vi "WriteControl2MCU.vi"(6 "error in (no error)":errorcluster, 8 "Config":T1, 9 "Control Code":u8 format="%.0x") -> (0 "error out":errorcluster)   [LabVIEW 2016]
uses:
  Settings/Settings.ctl
  Logging/Logging Configuration.ctl
  Hardware Configuration.ctl
  <vilib>/NI Modbus.llb/MB Serial Master Query Write Multiple Coils (poly).vi
  Acquisition.lvlib
  Logging/Logging.lvlib
  Settings/Settings.lvlib
panel:
  out "Exception Code":u8 format="%.0x"
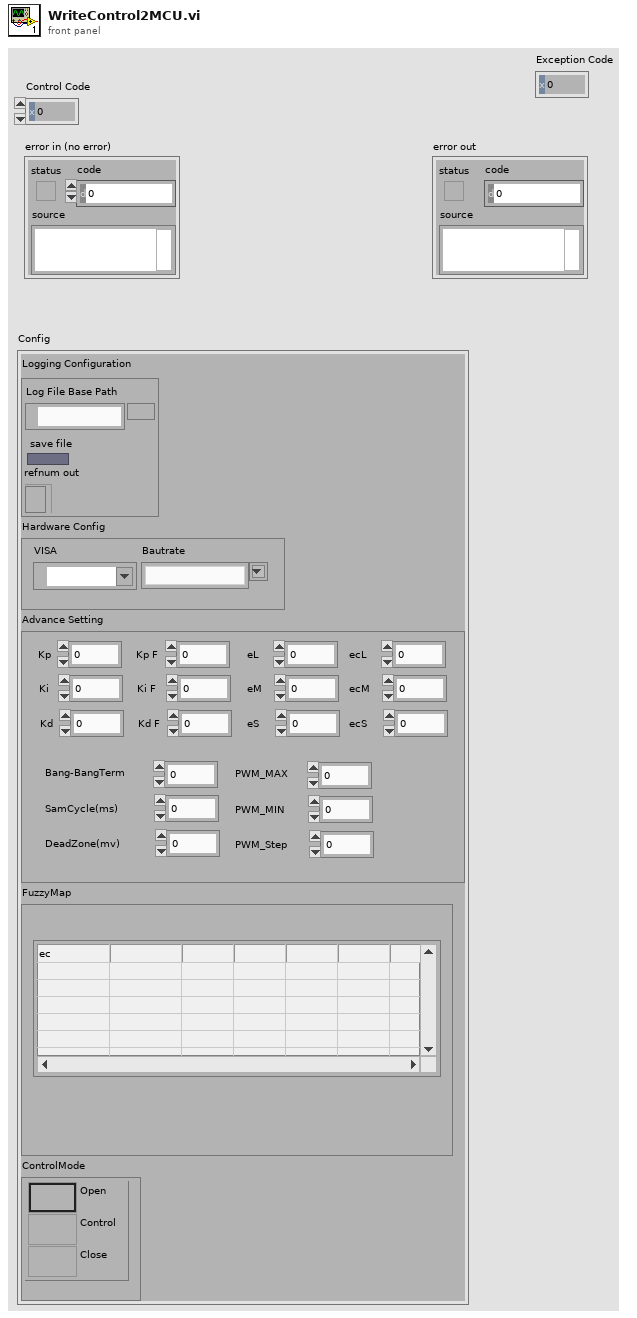
[diagram p1: front panel]
types:
  T1 = typedef "Settings.lvlib/Settings.ctl" = cluster{"Logging Configuration":T2, "Hardware Config":cluster{"Bautrate":string, "VISA":T3}, "Advance Setting":cluster{"PWM_Step":dbl, "PWM_MIN":dbl, "PWM_MAX":dbl, "DeadZone(mv)":dbl, "SamCycle(ms)":dbl, "Bang-BangTerm":dbl, "ecS":dbl, "ecM":dbl, "ecL":dbl, "eS":dbl, "eM":dbl, "eL":dbl, "Kd F":dbl, "Ki F":dbl, "Kp F":dbl, "Kd":dbl, "Ki":dbl, "Kp":dbl}, "FuzzyMap":cluster{"Table":string[][]}, "ControlMode":cluster{"Control":enum32{"1", "2", "4"}}}
  T2 = typedef "Logging.lvlib/Logging Configuration.ctl" = cluster{"Log File Base Path":path, "save file":bool, "refnum out":refnum<file>}
  T3 = typedef "Acquisition.lvlib/Hardware Configuration.ctl" = refnum<visa-resource-name>
  T4 = cluster{"Mode":enum16{"RTU", "ASCII"}, "Slave Address":u8}
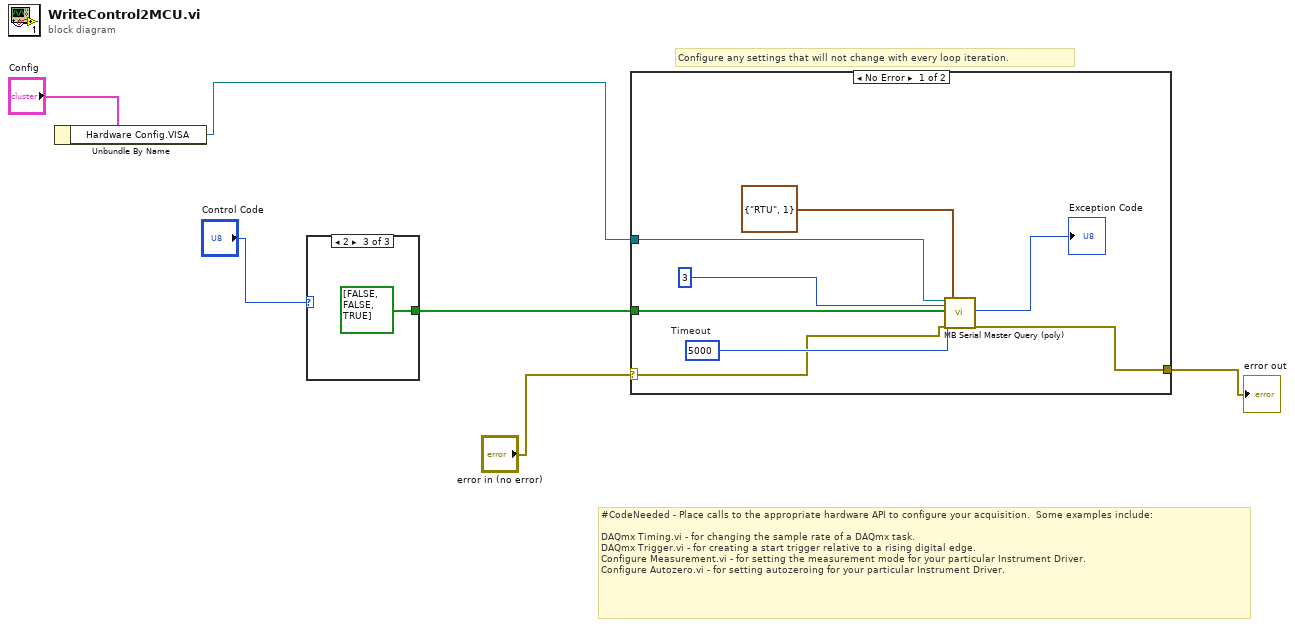
[diagram p0: block diagram]
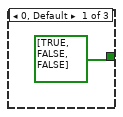
[diagram p2: hidden frame]
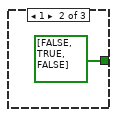
[diagram p3: hidden frame]
diagram:
  # "Configure any settings that will not change with every loop iteration."
  # "#CodeNeeded - Place calls to the appropriate hardware API to configure your acquisition.  Some examples include:\n\nDAQmx Timing.vi - for changing the sample rate of a DAQmx task.\nDAQmx Trigger.vi - for creating a start trigger relative to a rising digital edge.\nConfigure Measurement.vi - for setting the measurement mode for your particular Instrument Driver.\nConfigure Autozero.vi - for setting autozeroing for your particular Instrument Driver."
  n1 = Unbundle By Name("Config") -> ("Hardware Config.VISA"=w5:T3)
  n2 = case shown="2" "Control Code" {
    tunnel: [bool[] [TRUE, FALSE, FALSE] ("Coils") bool[] [FALSE, TRUE, FALSE] ("Coils") bool[] [FALSE, FALSE, TRUE] ("Coils")] -> w1
    frame 0, Default {
    }
    frame 1 {
    }
    frame 2 {
    }
  }
  n3 = case shown="No Error" "error in (no error)" {
    selector: "error in (no error)" -> [w12 w18]
    tunnel: w5 -> [w17 _]
    tunnel: [w11 w18] -> w3
    tunnel: w1 -> [w10 _]
    frame No Error {
      w15 = u32 5000  # Timeout
      n4 = call-poly <vilib>:"MB Serial Master Query (poly).vi"("VISA resource name"=w17, "Starting Address"=u16 3, "Coils"=w10, "Timeout"=w15, "error in"=w12, "Serial Parameters"=T4 {"Mode"=enum."RTU", "Slave Address"=1}) -> ("Exception Code"=→"Exception Code":u8, "error out"=w11:errorcluster)  [unwired: 11 in, 1 out]
    }
    frame Error {
    }
  }
  "error out" <- w3
